vi "write_check_input.vi"(8 "error in (no error)":errorcluster, 10 "check_input":bool=TRUE, 11 "IncrementalPCA in":refnum<class "IncrementalPCA.lvclass">) -> (0 "error out":errorcluster, 3 "IncrementalPCA out":refnum<class "IncrementalPCA.lvclass">)   [LabVIEW 2020, in "IncrementalPCA.lvclass"]
uses:
  IncrementalPCA.lvclass
  IncrementalPCA.lvclass/IncrementalPCA.ctl
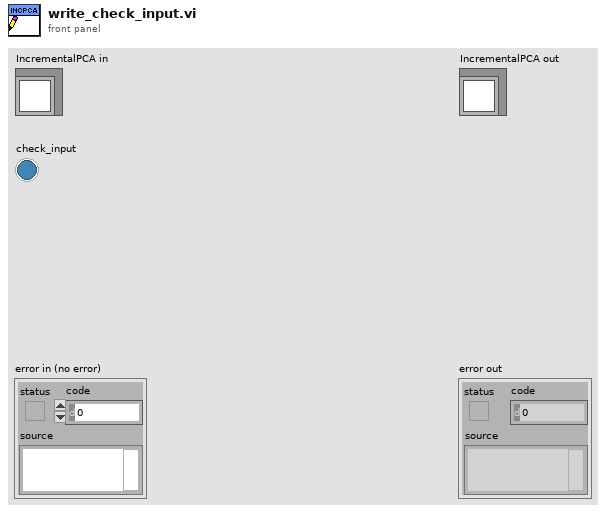
[diagram p1: front panel]
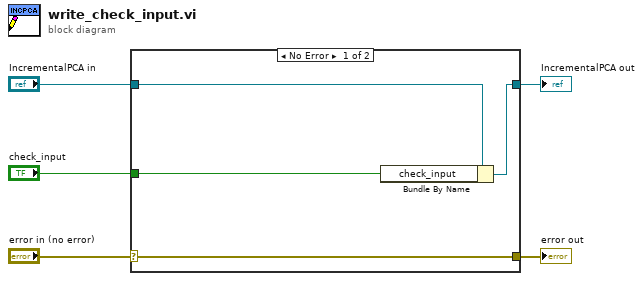
[diagram p0: block diagram]
diagram:
  n1 = case shown="No Error" "error in (no error)" {
    selector: "error in (no error)" -> [w9 w10]
    tunnel: [w9 w10] -> w4
    tunnel: [w7 w11] -> w2
    tunnel: "IncrementalPCA in" -> [w8 w11]
    tunnel: "check_input" -> [w6 _]
    frame No Error {
      n2 = Bundle By Name(cluster=w8, "check_input"=w6) -> (w7:refnum<class "IncrementalPCA.lvclass">)
    }
    frame Error {
    }
  }
  "error out" <- w4
  "IncrementalPCA out" <- w2
